vi "AIT_MER.vi"() -> ()   [LabVIEW 2014]
panel:
  out "String 3":string
  out "Temp C":dbl(slide) scale=-50.0..300.0
  out "String 2":string
  in  "Temp F":dbl(slide) scale=-299.0..900.0
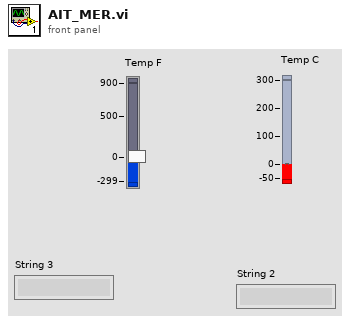
[diagram p1: front panel]
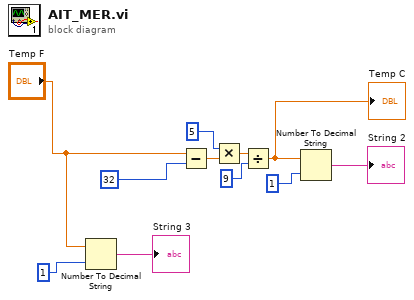
[diagram p0: block diagram]
diagram:
  n1 = Number To Decimal String(number="Temp F", width (-)=1) -> (decimal integer string=→"String 3":string)
  n2 = Subtract(x="Temp F", y=32) -> (x-y=w7:dbl)
  n3 = Multiply(x=5, y=w7) -> (x*y=w10:dbl)
  n4 = Divide(x=w10, y=9) -> (x/y=w4:dbl)
  "Temp C" <- w4
  n5 = Number To Decimal String(number=w4, width (-)=1) -> (decimal integer string=→"String 2":string)
